vi "Dpc Enable Pin Io.vi"(8 "error in (no error)":errorcluster, 9 "ptrid":u16, 10 "perc":i32, 11 "hif":u32) -> (0 "error out":errorcluster, 1 "ptrid out":u16, 2 "perc out":i32, 3 "hif out":u32, 5 "function return":i32)   [LabVIEW 2011, in "LVH-Adept.lvlib" / "DPCUTIL.lvlib"]
doc: "DPCAPI BOOL DpcEnablePinIo(HANDLE hif, ERC * perc, TRID * ptrid);"
uses:
  DPCUTIL.lvlib
  Resources/dpcutil.dll
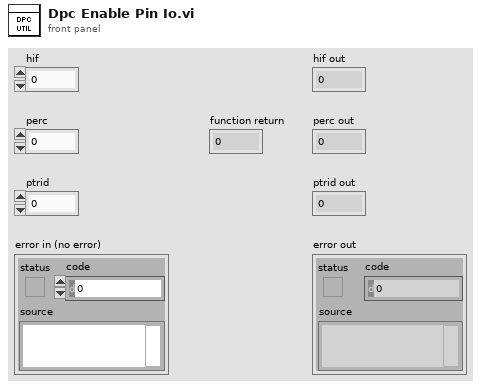
[diagram p1: front panel]
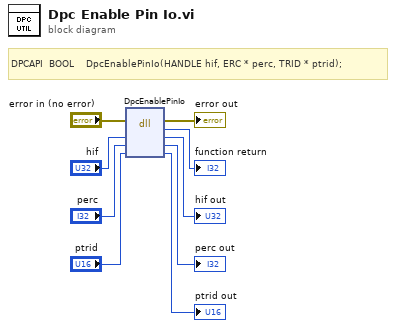
[diagram p0: block diagram]
diagram:
  # "DPCAPI  BOOL    DpcEnablePinIo(HANDLE hif, ERC * perc, TRID * ptrid);"
  n1 = dll-call lib="C:/github/labviewhacker/LVH-Adept/LabVIEW/vi.lib/LabVIEW Hacker/Adept/Private/Resources/dpcutil.*" fn="DpcEnablePinIo"(error in="error in (no error)", "hif"="hif", "perc"="perc", "ptrid"="ptrid") -> (error out=→"error out":errorcluster, →"function return":i32, "hif"=→"hif out":u32, "perc"=→"perc out":i32, "ptrid"=→"ptrid out":u16)  [unwired: 2 in, 1 out]
